vi "Desired vector (SubVI).vi"(4 "error in":errorcluster, 5 "v":dbl, 6 "R_p":dbl[][](array[numeric]), 7 "p":dbl) -> (0 "error out":errorcluster, 1 "p_ddot":dbl[](array[numeric]), 3 "p_d":dbl[](array[numeric]))   [LabVIEW 2014]
uses:
  <vilib>/imath/engines/lvmath2/RunTimeEngine/ArithmeticOperatorToken/NIMS_ArithmeticOperator_multmx(M,CV).vi
  <instcachedir>/0/NIMS_ArithmeticOperator_multmx(M,CV)_787B4652E60B4C52835A7FB23671E425.lvgen/NIMS_ArithmeticOperator_multmx(M,CV)_787B4652E60B4C52835A7FB23671E425_003.vi
  <vilib>/imathl/engines/lvmath/Functions/Error Handling/Create Error.vi
  <vilib>/imath/engines/lvmath2/RunTimeEngine/NodeEndStatement/NIMS_NodeEndStatement_Get Vector.vi
  <instcachedir>/0/NIMS_NodeEndStatement_Get Vector_00D1625602D843AD9D7EC134A9EC13A2.lvgen/NIMS_NodeEndStatement_Get Vector_00D1625602D843AD9D7EC134A9EC13A2_001.vi
  <vilib>/imath/engines/lvmath/Functions/Error Handling/MergeErrorsWrapper.vi
  <vilib>/imath/engines/lvmath2/RunTimeEngine/NodeEndStatement/NIMS_NodeEndStatement_Output.vi
  <instcachedir>/0/NIMS_NodeEndStatement_Output_53EC0D466D134D7ABD903AC30B43404B.lvgen/NIMS_NodeEndStatement_Output_53EC0D466D134D7ABD903AC30B43404B_005.vi
  <vilib>/imath/engines/lvmath2/RunTimeEngine/ErrorHandling/NIMS_Finalize Error.vi
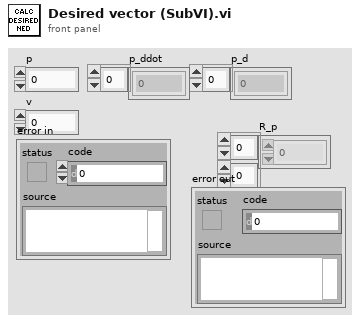
[diagram p1: front panel]
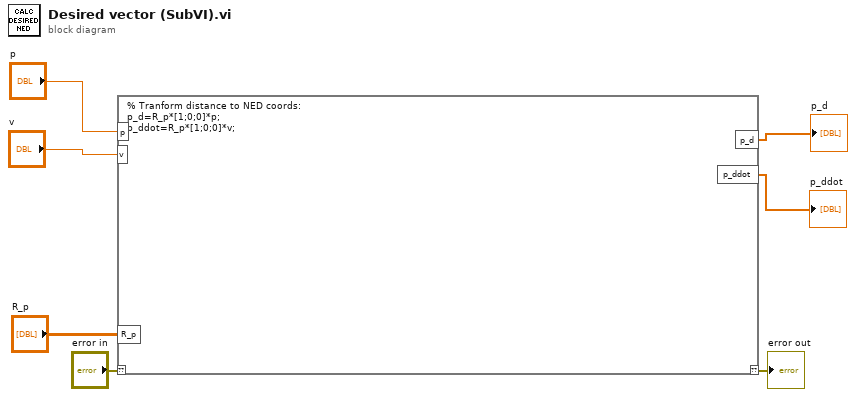
[diagram p0: block diagram]
diagram:
  n1 = mathscript code="% Tranform distance to NED coords:\np_d=R_p*[1;0;0]*p;\np_ddot=R_p*[1;0;0]*v;"("??"="error in", "p"="p", "R_p"="R_p", "v"="v") -> ("??"=→"error out":errorcluster, "p_d"=→"p_d":dbl[], "p_ddot"=→"p_ddot":dbl[])
